vi "Actor Core.vi"(8 "error in":errorcluster, 11 "Timer test in":refnum<class "Timer test.lvclass">) -> (0 "error out":errorcluster, 3 "Actor out":refnum<class "Actor.lvclass">)   [LabVIEW 2015, in "Timer test.lvclass"]
doc: "(<B>Filename</B>: Actor Framework.lvlib:Actor.lvclass:Actor Core.vi)\n\nReceives messages to the actor, reacts to them, and initiates any error handling that may shut the actor down.\n\nDescendant classes may override this VI to append parallel tasks for the actor to complete while it handles messages. Overrides use the Call Parent Method node."
uses:
  Timer test.lvclass
  <vilib>/ActorFramework/Actor/Actor.lvclass
  Log time.ctl
  Timer test.lvclass/Timer test.ctl
  Mag Lab Root/Mag Lab Root.lvclass/Mag Lab Root.ctl
  <vilib>/ActorFramework/Actor/Actor.lvclass/Actor.ctl
  <vilib>/ActorFramework/Message Enqueuer/Message Enqueuer.lvclass/Message Enqueuer.ctl
  Measurement Timer.lvclass
  Measurement Timer.lvclass/Measurement Timer.ctl
  Mag Lab Measure Base Messages/Launch Nested Object Msg/Launch Nested Object Msg.lvclass/Launch Nested Object Msg.ctl
  Mag Lab Root Messages/Recieve Request for Result Msg/Recieve Request for Result Msg.lvclass/Recieve Request for Result Msg.ctl
  Write millisecond multiple.vi
  Write Time Reference.vi
  <vilib>/ActorFramework/Message Enqueuer/Init from Existing Queue.vi
  <vilib>/ActorFramework/Message Enqueuer/Enqueue.vi
  <vilib>/ActorFramework/Message Priority Queue/Priority Enqueue.vi
  Mag Lab Measure Controller/Mag Lab Measure Controller.lvclass
  <vilib>/ActorFramework/Message Enqueuer/Message Enqueuer.lvclass
  <vilib>/ActorFramework/Stop Msg/Stop Msg.lvclass
  Mag Lab Measure Base Messages/Launch Nested Object Msg/Launch Nested Object Msg.lvclass
  Mag Lab Root Messages/Recieve Request for Result Msg/Recieve Request for Result Msg.lvclass
  Mag Lab Root/Mag Lab Root.lvclass
  Mag Lab Error Handler/Mag Lab Error Handler.lvclass
panel:
  in  "Time reference":T1
  in  "Timer name":string="A"
  in  "millisecond multiple":u32=1000
  in  "Add Timer":bool
  in  "Log":string
  in  "Stop Button":bool
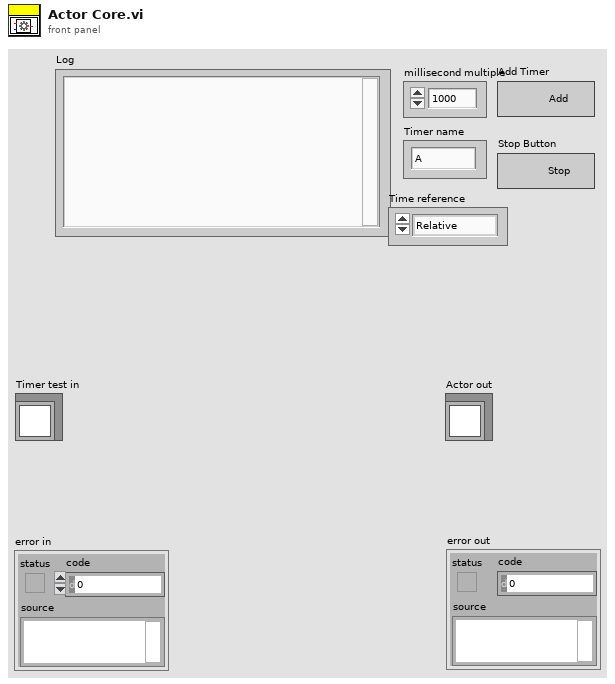
[diagram p1: front panel]
types:
  T1 = typedef "Log time.ctl" = enum16{"Relative", "Absolute", "Do not log"}
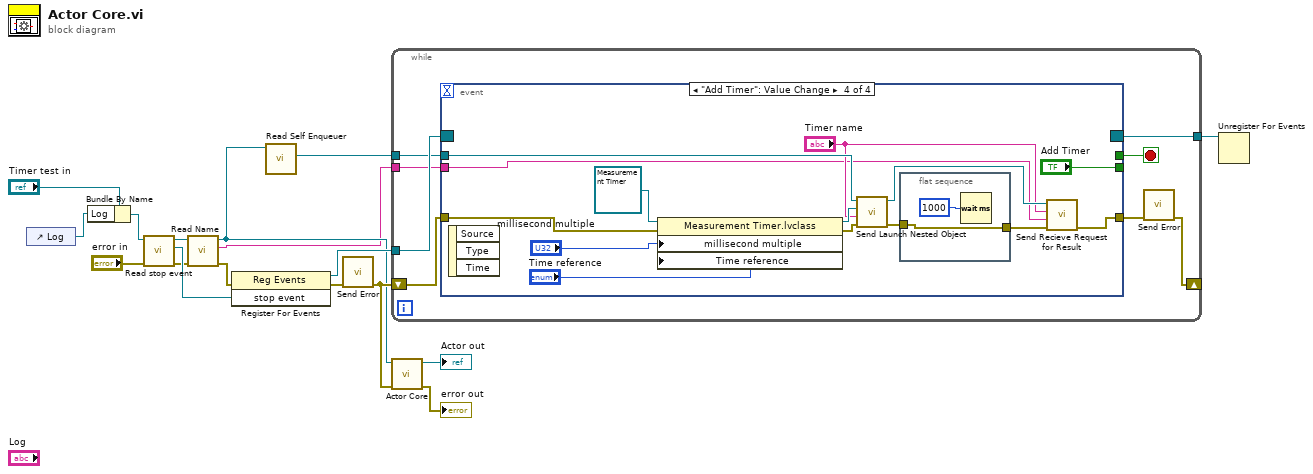
[diagram p0: block diagram]
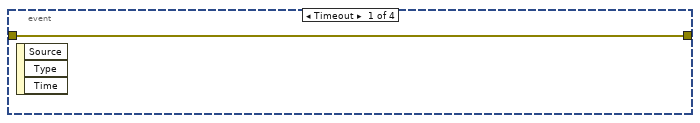
[diagram p2: hidden frame]
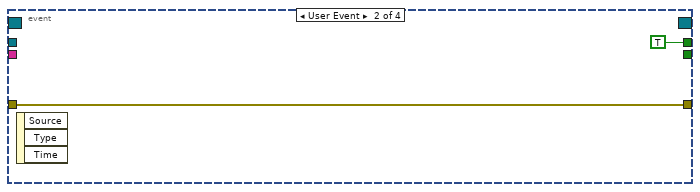
[diagram p3: hidden frame]
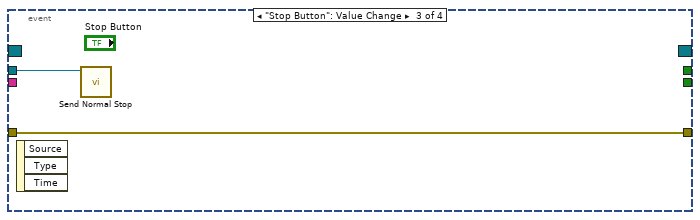
[diagram p4: hidden frame]
diagram:
  n1 = control-ref of="Log"() -> (w7:refnum<vi>)
  n2 = Bundle By Name(cluster="Timer test in", "Log"=w7) -> (w8:refnum<class "Timer test.lvclass">)
  n3 = call "Read stop event.vi"("error in (no error)"="error in", "Mag Lab Root in"=w8) -> ("error out"=w3:errorcluster, "stop event"=w14:refnum<user-event>, "Mag Lab Root out"=w5:refnum<class "Timer test.lvclass">)  [unwired: 7 in]
  n4 = call "Read Name.vi"("error in (no error)"=w3, "Mag Lab Root in"=w5) -> ("error out"=w2:errorcluster, "Name"=w1:string, "Mag Lab Root out"=w4:refnum<class "Timer test.lvclass">)  [unwired: 7 in]
  n5 = register-events(error in=w2, w14) -> (reference out=w12:refnum<event-registration>, error out=w13:errorcluster)  [unwired: 1 in]
  n6 = call <vilib>:"Read Self Enqueuer.vi"("Actor"=w4) -> ("Self Enqueuer"=w10:refnum<class "Message Enqueuer.lvclass">)  [unwired: 10 in]
  n7 = call "Send Error.vi"("error in (no error)"=w13) -> ("error out"=w6:errorcluster)  [unwired: 9 in, 1 out]
  n8 = while {
    tunnel: w12 -> [w25]
    tunnel: [w24] -> w11
    tunnel: w10 -> [w22]
    shift-right: [w19] -> _
    shift-left: w6 -> [w21]
    tunnel: w1 -> [w18]
    stop <- w23 stop-if-true
    n9 = event shown="[3] \"Add Timer\": Value Change" {
      selector: w25 -> [_ _ _ _]
      dyn-events: [_ _ _ _] -> w24
      timeout: _ -> [_ _ _ _]
      tunnel: [_ TRUE _ _] -> w23
      tunnel: w22 -> [_ _ w30 w43]
      tunnel: [_ _ _ "Add Timer"] -> _
      tunnel: w21 -> [w26 w27 w29 w38]
      tunnel: [w26 w27 w29 w36] -> w20
      tunnel: w18 -> [_ _ _ w32]
      event Timeout {
        n10 = event-data() -> ()  [unwired: 1 in, 3 out]
      }
      event User Event {
        n11 = event-data() -> ()  [unwired: 1 in, 3 out]
      }
      event "Stop Button": Value Change {
        n12 = event-data() -> ()  [unwired: 1 in, 3 out]
        n13 = call <vilib>:"Send Normal Stop.vi"("Message Enqueuer"=w30) -> ()  [unwired: 10 in, 1 out]
      }
      event "Add Timer": Value Change {
        n14 = event-data() -> ()  [unwired: 1 in, 3 out]
        n15 = property class="Measurement Timer.lvclass"(reference=refnum<class "Measurement Timer.lvclass"> refnum ("Measurement Timer.lvclass"), error in=w38, "millisecond multiple"="millisecond multiple", "Time reference"="Time reference") -> (reference out=w41:refnum<class "Measurement Timer.lvclass">, error out=w39:errorcluster)
        n16 = call "Send Launch Nested Object.vi"("error in (no error)"=w39, "name"="Timer name", "Object"=w41, "Message Enqueuer"=w43) -> ("error out"=w35:errorcluster, "Message Enqueuer out"=w37:refnum<class "Message Enqueuer.lvclass">)  [unwired: 6 in]
        n17 = flat-sequence {
          tunnel: w35 -> [w46]
          tunnel: [w46] -> w34
          frame #0 {
            n18 = Wait (ms)(milliseconds to wait=u32 1000) -> ()  [unwired: 1 out]
          }
        }
        n19 = call "Send Recieve Request for Result.vi"("error in (no error)"=w34, "Requestor"=w32, "Requestee"="Timer name", "Message Enqueuer"=w37) -> ("error out"=w36:errorcluster)  [unwired: 6 in, 1 out]
      }
    }
    n20 = call "Send Error.vi"("error in (no error)"=w20) -> ("error out"=w19:errorcluster)  [unwired: 9 in, 1 out]
  }
  n21 = call-parent "Actor Core.vi"("error in"=w6, "Mag Lab Measure Base in"=w4) -> ("error out"=→"error out":errorcluster, "Actor out"=→"Actor out":refnum<class "Actor.lvclass">)  [unwired: 8 in]
  n22 = Unregister For Events(event registration refnum=w11) -> ()  [unwired: 1 in, 1 out]
